vi "Get Section CD Item Property Values.vi"(8 "error in (no error)":errorcluster, 10 "Group name":string, 11 "CD Parameter Manager in":refnum<class "CD Parameter Manager.lvclass">) -> (0 "error out":errorcluster, 3 "CD Parameter Manager out":refnum<class "CD Parameter Manager.lvclass">)   [LabVIEW 2019, in "CD Parameter Manager API.lvlib" / "CD Parameter Manager.lvclass"]
uses:
  CD Parameter Manager.lvclass
  CD Parameter Manager.lvclass/CD Parameter Manager.ctl
  Parameter Class/Parameter.lvclass
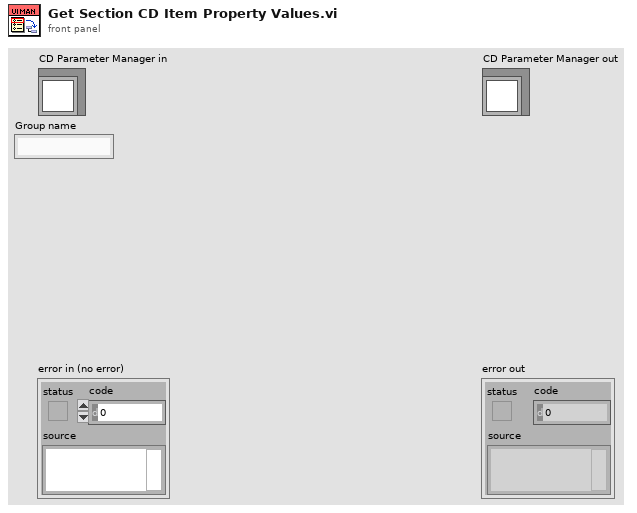
[diagram p1: front panel]
types:
  T1 = cluster{"Group name":string, "Controls":refnum<class "Parameter.lvclass">[]}[]
  T2 = typedef "Custom Device API.lvlib/Custom Device Item Ref.ctl" = u64
  T3 = cluster{"Group name":string, "Controls":refnum<class "Parameter.lvclass">[]}
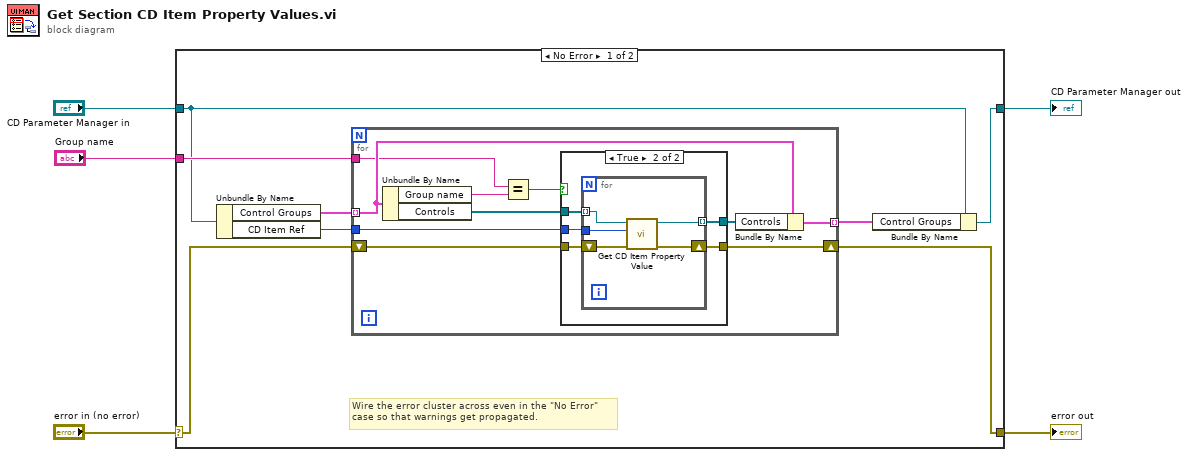
[diagram p0: block diagram]
diagram:
  n1 = case shown="No Error" "error in (no error)" {
    selector: "error in (no error)" -> [w10 w37]
    tunnel: [w9 w37] -> w4
    tunnel: [w8 w36] -> w2
    tunnel: "CD Parameter Manager in" -> [w6 w36]
    tunnel: "Group name" -> [w7 _]
    frame No Error {
      # "Wire the error cluster across even in the \"No Error\"\ncase so that warnings get propagated."
      n2 = Unbundle By Name(w6) -> ("Control Groups"=w13:T1, "CD Item Ref"=w12:T2)
      n3 = for {
        tunnel: w13 -> [w19] mode=indexing
        tunnel: w12 -> [w22]
        shift-right: [w21] -> w9
        shift-left: w10 -> [w23]
        tunnel: [w17] -> w11 mode=indexing
        tunnel: w7 -> [w15]
        n4 = Unbundle By Name(w19) -> ("Group name"=w16:string, "Controls"=w20:refnum<class "Parameter.lvclass">[])
        n5 = Equal?(x=w15, y=w16) -> (x = y?=w14:bool)
        n6 = case shown="True" w14 {
          tunnel: w23 -> [w25 w30]
          tunnel: w22 -> [_ w29]
          tunnel: [w25 w28] -> w21
          tunnel: w20 -> [w24 w27]
          tunnel: [w24 w26] -> w18
          frame False {
          }
          frame True {
            n7 = for {
              tunnel: w29 -> [w34]
              shift-right: [w33] -> w28
              shift-left: w30 -> [w35]
              tunnel: [w32] -> w26 mode=indexing
              tunnel: w27 -> [w31] mode=indexing
              n8 = call-dynamic "Get CD Item Property Value.vi"("error in (no error)"=w35, "CD Item Ref in"=w34, "Parameter in"=w31) -> ("error out"=w33:errorcluster, "Parameter out"=w32:refnum<class "Parameter.lvclass">)  [unwired: 7 in]
            }
          }
        }
        n9 = Bundle By Name(cluster=w19, "Controls"=w18) -> (w17:T3)
      }
      n10 = Bundle By Name(cluster=w6, "Control Groups"=w11) -> (w8:refnum<class "CD Parameter Manager.lvclass">)
    }
    frame Error {
    }
  }
  "error out" <- w4
  "CD Parameter Manager out" <- w2
